vi "Exout.vi"(5 "IN VARIANT":variant, 7 "ip":string, 9 "Name in":string) -> (10 "Operation Ok":bool)   [LabVIEW 2015]
uses:
  LI_states.ctl
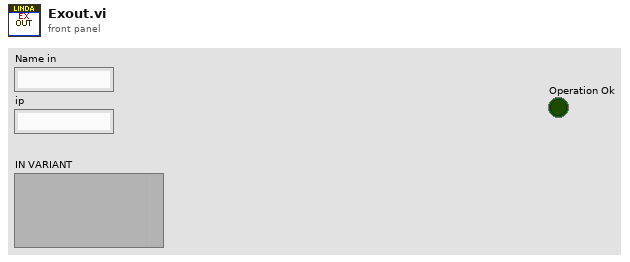
[diagram p1: front panel]
types:
  T1 = typedef "LI_states.ctl" = enum16{"Out", "In", "Rd", "Inp", "Rdp", "Init", "Cleanup", "RdAll"}
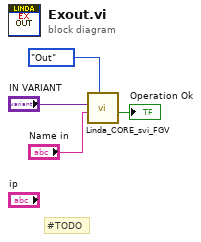
[diagram p0: block diagram]
diagram:
  # "#TODO"
  n1 = call "Linda_CORE_svi_FGV.vi"("OP"=LI_states."Out", "Name in"="Name in", "IN VARIANT"="IN VARIANT") -> ("Valid Op"=→"Operation Ok":bool)  [unwired: 5 in, 3 out]
